vi "Page_Info_Read.vi"(6 "ctlReferences":T1, 8 "error in (no error)":errorcluster, 11 "AB_Targetfile in":refnum<class "AB_Targetfile.lvclass">) -> (0 "error out":errorcluster, 3 "AB_Targetfile out":refnum<class "AB_Targetfile.lvclass">)   [LabVIEW 2020, in "AB_Targetfile.lvclass"]
uses:
  <vilib>/AppBuilder/AB_Classes/TargetFile/AB_Targetfile.lvclass
  <resource>/Framework/Providers/Builds/AppBuilder/AB_UI_Page_Info_References.ctl
  <vilib>/AppBuilder/AB_Classes/TargetFile/AB_Targetfile.lvclass/AB_Targetfile.ctl
  <vilib>/AppBuilder/AB_Classes/Build/AB_Build.lvclass
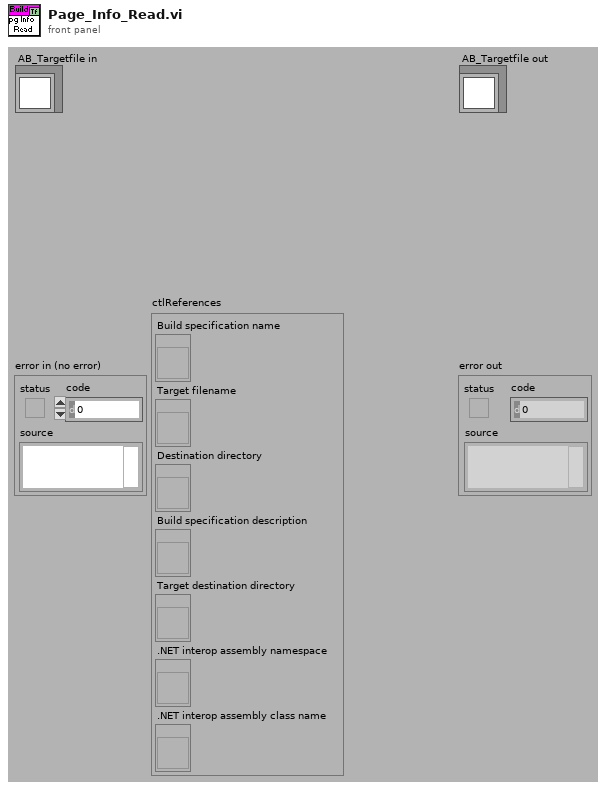
[diagram p1: front panel]
types:
  T1 = typedef "AB_UI_Page_Info_References.ctl" = cluster{"Build specification name":refnum<vi>, "Target filename":refnum<vi>, "Destination directory":refnum<vi>, "Build specification description":refnum<vi>, "Target destination directory":refnum<vi>, ".NET interop assembly namespace":refnum<vi>, ".NET interop assembly class name":refnum<vi>}
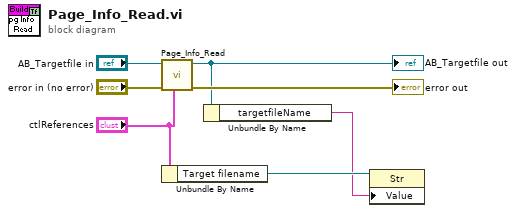
[diagram p0: block diagram]
diagram:
  n1 = call-parent "Page_Info_Read.vi"("ctlReferences"="ctlReferences", "error in (no error)"="error in (no error)", "AB_Build in"="AB_Targetfile in") -> ("error out"=→"error out":errorcluster, "AB_Build out"=w2:refnum<class "AB_Targetfile.lvclass">)  [unwired: 7 in]
  "AB_Targetfile out" <- w2
  n2 = Unbundle By Name("ctlReferences") -> ("Target filename"=w4:refnum<vi>)
  n3 = Unbundle By Name(w2) -> ("targetfileName"=w1:string)
  n4 = property class="Str"(reference=w4, "Value"=w1) -> ()  [unwired: 1 in, 2 out]
